vi "ListboxItems (SubVI).vi"(2 "error in (no error)":errorcluster, 3 "Clear":bool, 4 "MCListbox Refnum":refnum<vi>, 5 "path":path) -> (0 "error out":errorcluster)   [LabVIEW 2013, in "main.lvlib"]
uses:
  main.lvlib
  <vilib>/regexp/Match Regular Expression.xnode
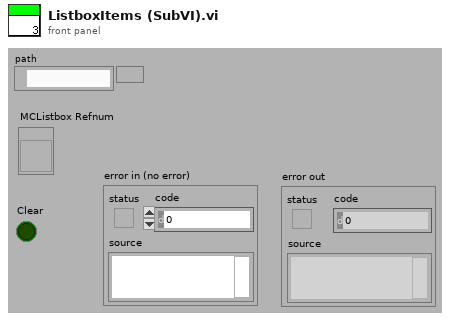
[diagram p1: front panel]
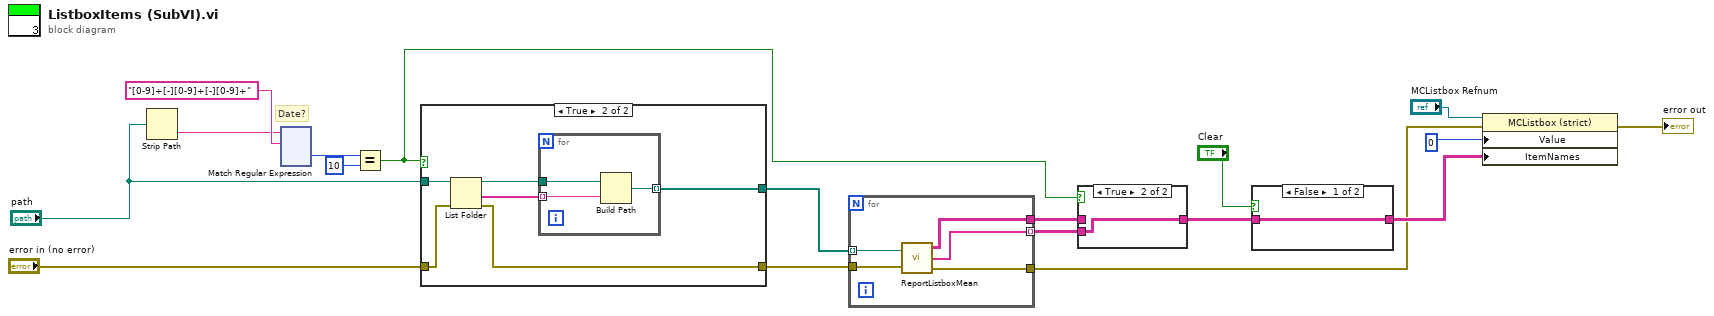
[diagram p0: block diagram]
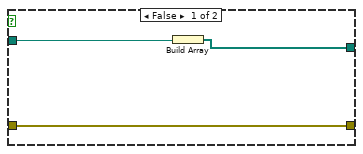
[diagram p3: hidden frame]
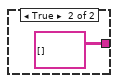
[diagram p4: hidden frame]
diagram:
  # "Date?"
  n1 = Strip Path(path="path") -> (name=w3:string)  [unwired: 1 out]
  n2 = xnode "Match Regular Expression"("input string"=w3, "regular expression"="[0-9]+[-][0-9]+[-][0-9]+") -> ("offset past match"=w12:i32)  [unwired: 4 in, 4 out]
  n3 = Equal?(x=w12, y=10) -> (x = y?=w2:bool)
  n4 = case shown="True" w2 {
    tunnel: "path" -> [w20 w27]
    tunnel: "error in (no error)" -> [w21 w26]
    tunnel: [w21 w25] -> w9
    tunnel: [w19 w22] -> w8
    frame False {
      n5 = Build Array(w20) -> (w19:path[])
    }
    frame True {
      n6 = List Folder(path=w27, error in=w26) -> (path out=w24:path, folder names=w23:string[], error out=w25:errorcluster)  [unwired: 2 in, 1 out]
      n7 = for {
        tunnel: w24 -> [w30]
        tunnel: w23 -> [w29] mode=indexing
        tunnel: [w28] -> w22 mode=indexing
        n8 = Build Path(base path=w30, name or relative path=w29) -> (appended path=w28:path)
      }
    }
  }
  n9 = for {
    tunnel: w9 -> [w35]
    tunnel: [w34] -> w6
    tunnel: [w33] -> w4
    tunnel: w8 -> [w32] mode=indexing
    tunnel: [w31] -> w7 mode=indexing
    n10 = call "ReportListboxMean.vi"("error in (no error)"=w35, "path"=w32) -> ("error out"=w33:errorcluster, "Means"=w31:string[], "Output Array"=w34:string[][])
  }
  n11 = case shown="True" w2 {
    tunnel: w7 -> [_ w37]
    tunnel: w6 -> [w36 _]
    tunnel: [w36 w37] -> w5
    frame False {
    }
    frame True {
    }
  }
  n12 = case shown="False" "Clear" {
    tunnel: [w38 string[][] [] ("Item Names")] -> w16
    tunnel: w5 -> [w38 _]
    frame False {
    }
    frame True {
    }
  }
  n13 = property class="MCListbox (strict)"(reference="MCListbox Refnum", error in=w4, "Value"=0, "ItemNames"=w16) -> (error out=→"error out":errorcluster)  [unwired: 1 out]
